vi "Fail interlock.vi"(6 "Select":bool, 7 "Command":T1(ring)=enum."Write task", 8 "error in":errorcluster caption="err out", 9 "Fail Index Out":bool[](array[boolean]), 10 "Inter lock":bool, 11 "Pause":refnum<vi>) -> (0 "error out":errorcluster caption="err out")   [LabVIEW 2016]
uses:
  <vilib>/DAQmx/write.llb/DAQmx Write (Digital Bool 1Line 1Point).vi
  <vilib>/DAQmx/create/channels.llb/DAQmx Create Channel (DO-Digital Output).vi
  <vilib>/DAQmx/miscellaneous.llb/DAQmx Fill In Error Info.vi
panel:
  out "task out":refnum<k21>
  out "Flag":bool=TRUE
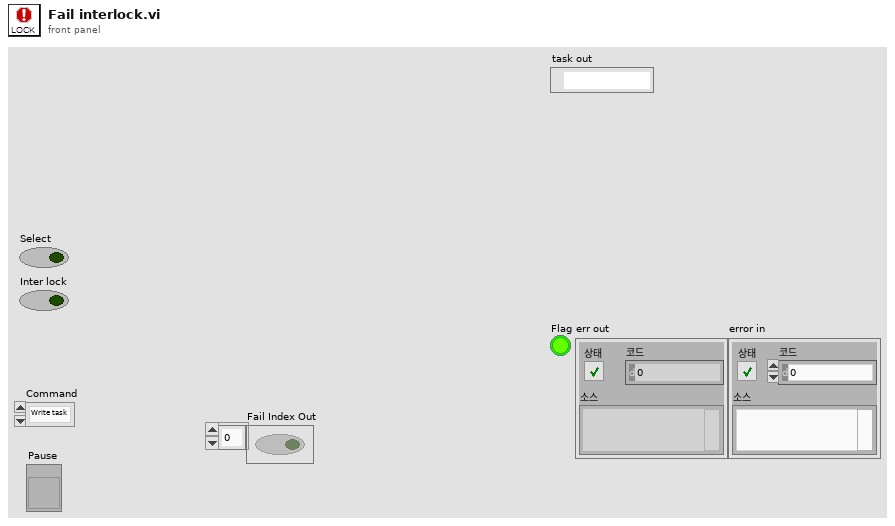
[diagram p1: front panel]
types:
  T1 = enum16{"Flag", "Write task", "Select Data", "Init"}
  T2 = cluster{"Test Information":cluster{"date":string, "custom":string, "oper":string, "package":string, "pkg side":string, "solder":string, "brd side":string, "paste":string, "reflow":string}, "Sensor Set":cluster{"Accelerometer":cluster{"Sensitivity(mV/g)":dbl}, "Strain Guage":cluster{"Ch.":dbl[], "Gage factor":dbl[], "Resistance":dbl[], "Poisson ratio":dbl[]}}, "Resistor Set":cluster{"Criterion Level":dbl, "Res. Set":cluster{"Res. Ch":dbl, "Res. Active":bool, "Res Initial":dbl}[]}, "Test Stop Condition":cluster{"Test cycle":u16, "Fail number in a cycle":u16, "Fail factor":cluster{"Duration":u16, "Fail No.":u16}}, "Acceleration Condition ":cluster{"Shock duration pecent [%]":u16, "Filter cutoff freq":u32}, "Save":cluster{"Save Path":path, "File Name":string}}
  T3 = cluster{"Res. Ch":dbl, "Res. Active":bool, "Res Initial":dbl}[]
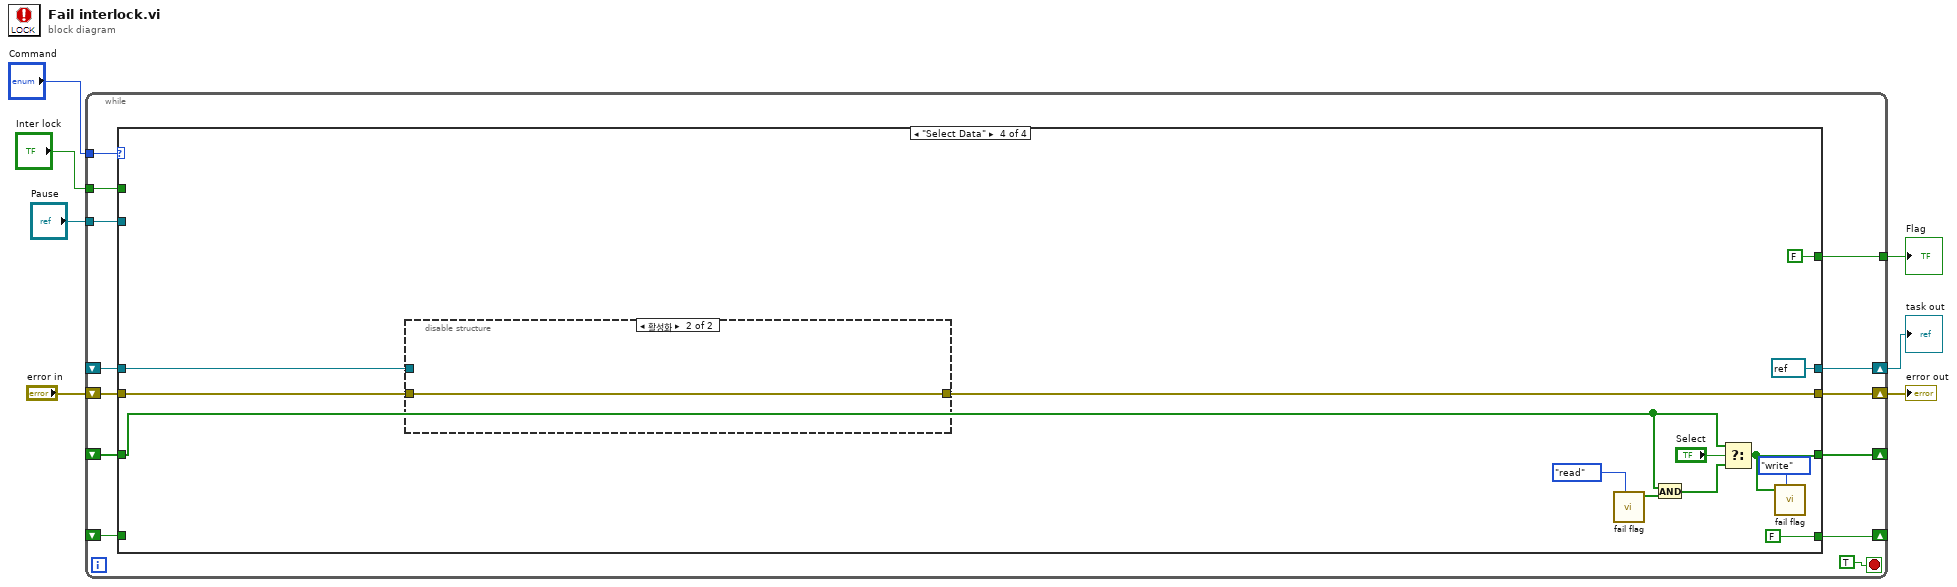
[diagram p0: block diagram]
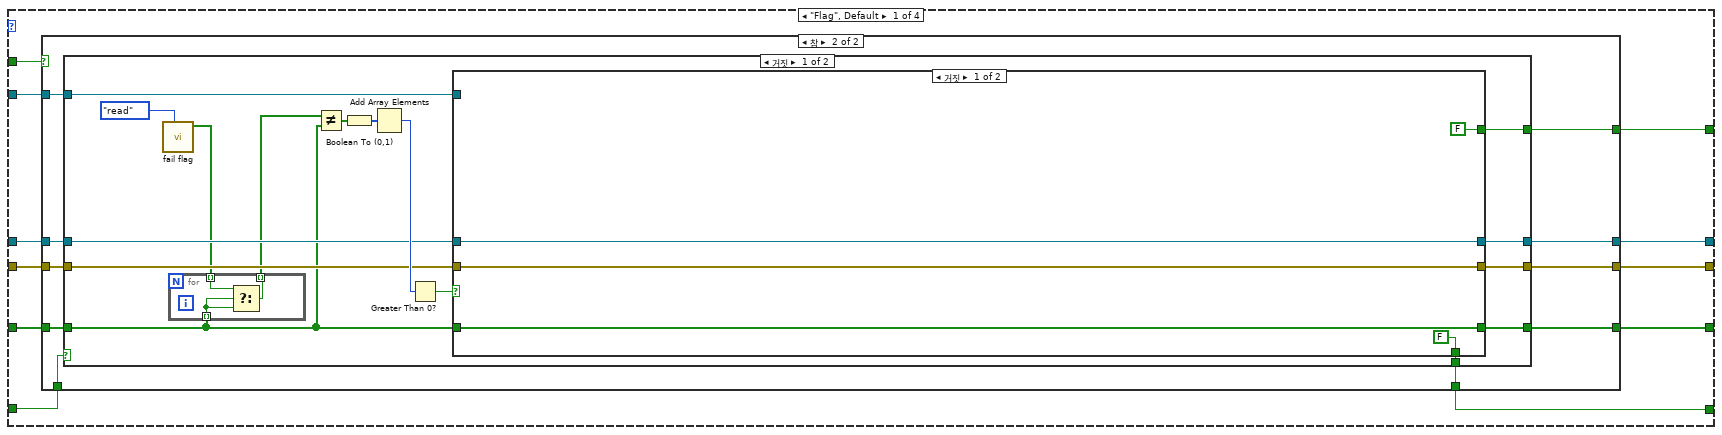
[diagram p2: hidden frame]
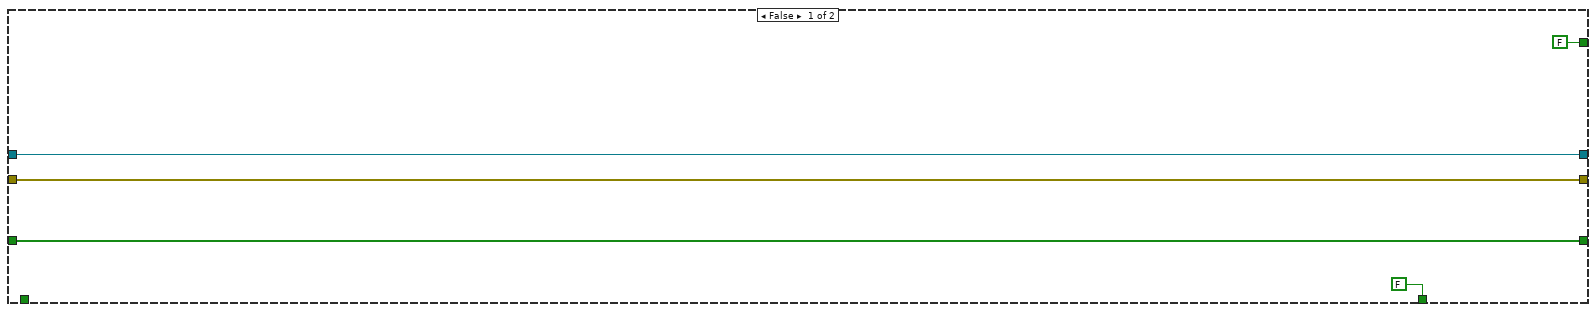
[diagram p3: hidden frame]
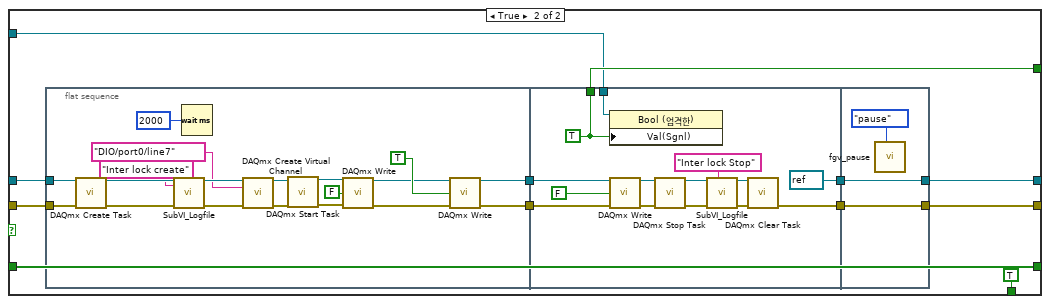
[diagram p4: hidden frame]
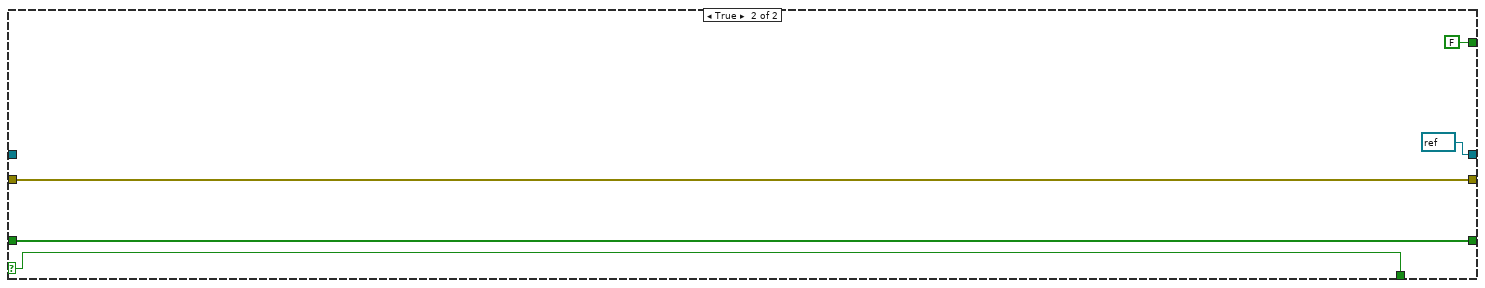
[diagram p5: hidden frame]
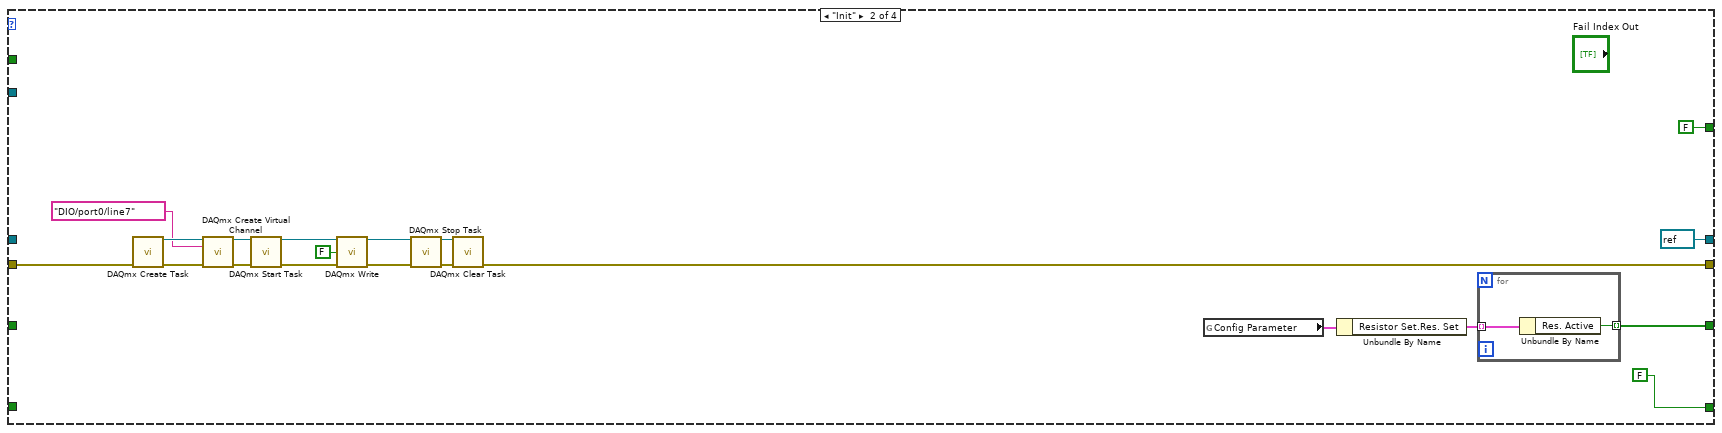
[diagram p6: hidden frame]
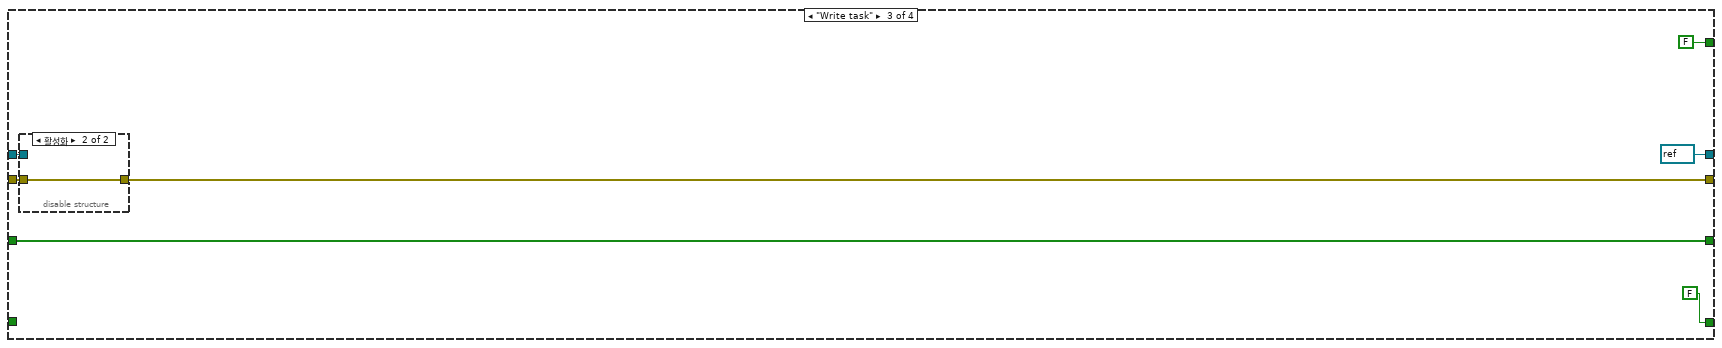
[diagram p7: hidden frame]
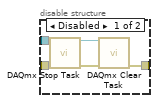
[diagram p8: hidden frame]
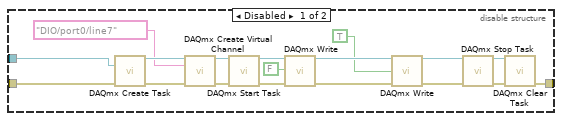
[diagram p9: hidden frame]
diagram:
  n1 = while {
    tunnel: "Command" -> [w19]
    shift-right: [w18] -> _
    shift-left: _ -> [w17]
    tunnel: [w16] -> w6
    tunnel: "Pause" -> [w15]
    shift-right: [w13] -> w1
    shift-left: _ -> [w14]
    shift-right: [w12] -> w4
    shift-left: "error in" -> [w11]
    tunnel: "Inter lock" -> [w10]
    shift-right: [w9] -> _
    shift-left: _ -> [w8]
    stop <- TRUE stop-if-true
    n2 = case shown="\"Select Data\"" w19 {
      tunnel: [w26 w134 w150 w157] -> w18
      tunnel: w17 -> [w27 _ w150 w160]
      tunnel: [w31 FALSE FALSE FALSE] -> w16
      tunnel: w15 -> [w30 _ _ _]
      tunnel: w14 -> [w29 _ w147 w166]
      tunnel: [w28 refnum<k21> refnum ("task out") refnum<k21> refnum ("task out") refnum<k21> refnum ("task out")] -> w13
      tunnel: [w23 w129 w145 w164] -> w12
      tunnel: w11 -> [w24 w137 w146 w165]
      tunnel: w10 -> [w25 _ _ _]
      tunnel: [w22 FALSE FALSE FALSE ("Res. Active")] -> w9
      tunnel: w8 -> [w21 _ _ _]
      frame "Flag", Default {
        n3 = case shown="참" w25 {
          tunnel: [FALSE w46] -> w31
          tunnel: w30 -> [_ w45]
          tunnel: w29 -> [w36 w41]
          tunnel: [w36 w44] -> w28
          tunnel: w27 -> [w35 w43]
          tunnel: [w35 w37] -> w26
          tunnel: w24 -> [w33 w40]
          tunnel: [w33 w42] -> w23
          tunnel: [FALSE w39] -> w22
          tunnel: w21 -> [_ w38]
          frame False {
          }
          frame True {
            n4 = case shown="거짓" w38 {
              selector: w38 -> [_ w118]
              tunnel: [w57 FALSE] -> w46
              tunnel: w45 -> [w56 _]
              tunnel: [w55 refnum<k21> refnum ("task out")] -> w44
              tunnel: w43 -> [w47 w117]
              tunnel: [w54 w119] -> w42
              tunnel: w41 -> [w53 _]
              tunnel: w40 -> [w52 w119]
              tunnel: [w51 w118] -> w39
              tunnel: [w50 w117] -> w37
              frame False {
                n5 = call "fail flag.vi"("Command"=enum16{"init", "read", "write"}."read") -> ("Fail Index Out"=w49:bool[])  [unwired: 10 in]
                n6 = for {
                  tunnel: w47 -> [w63] mode=indexing
                  tunnel: w49 -> [w65] mode=indexing
                  tunnel: [w64] -> w48 mode=indexing
                  n7 = Select(t=w65, s=w63, f=w63) -> (s? t:f=w64:bool)
                }
                n8 = Not Equal?(x=w48, y=w47) -> (x != y?=w61:bool[])
                n9 = Boolean To (0,1)(Boolean=w61) -> (0, 1=w60:i16[])
                n10 = Add Array Elements(numeric array=w60) -> (sum=w59:i16)
                n11 = Greater Than 0?(x=w59) -> (x > 0?=w58:bool)
                n12 = case shown="거짓" w58 {
                  tunnel: [w69 w79] -> w50
                  tunnel: [FALSE w72] -> w57
                  tunnel: w56 -> [_ w71]
                  tunnel: w53 -> [w66 w82]
                  tunnel: [w66 w81] -> w55
                  tunnel: w47 -> [w69 w79]
                  tunnel: w52 -> [w67 w78]
                  tunnel: [w67 w76] -> w54
                  tunnel: [FALSE TRUE] -> w51
                  frame False {
                  }
                  frame True {
                    n13 = flat-sequence {
                      tunnel: w82 -> [w93]
                      tunnel: [w100] -> w80
                      tunnel: w78 -> [w92]
                      tunnel: [w97] -> w77
                      tunnel: w80 -> [w112]
                      tunnel: w77 -> [w109]
                      tunnel: [refnum<k21> refnum ("task out")] -> w74
                      tunnel: [w106] -> w73
                      tunnel: [w105] -> w72
                      tunnel: w71 -> [w104]
                      tunnel: [w115] -> w76
                      tunnel: [w116] -> w81
                      tunnel: w74 -> [w116]
                      tunnel: w73 -> [w115]
                      frame #0 {
                        n14 = call <vilib>:"DAQmx Create Task.vi"("task to copy"=w93, "error in"=w92) -> ("task out"=w96:refnum<k21>, "error out"=w89:errorcluster)  [unwired: 12 in]
                        n15 = call "SubVI_Logfile.vi"("Title"="Inter lock create", "error in"=w89) -> ("error out"=w88:errorcluster)  [unwired: 9 in]
                        n16 = Wait (ms)(milliseconds to wait=u32 2000 ("대기 시간(ms)")) -> ()  [unwired: 1 out]
                        n17 = call-poly <vilib>:"DAQmx Create Virtual Channel.vi"("task in"=w96, "lines"=tag "DIO/port0/line7", "error in"=w88) -> ("task out"=w86:refnum<k21>, "error out"=w84:errorcluster)  [unwired: 11 in]
                        n18 = call <vilib>:"DAQmx Start Task.vi"("task/channels in"=w86, "error in"=w84) -> ("task out"=w85:refnum<k21>, "error out"=w83:errorcluster)  [unwired: 12 in]
                        n19 = call-poly <vilib>:"DAQmx Write.vi"("task/channels in"=w85, "data"=FALSE, "error in"=w83) -> ("task out"=w91:refnum<k21>, "error out"=w90:errorcluster)  [unwired: 10 in, 1 out]
                        n20 = call-poly <vilib>:"DAQmx Write.vi"("task/channels in"=w91, "data"=TRUE, "error in"=w90) -> ("task out"=w100:refnum<k21>, "error out"=w97:errorcluster)  [unwired: 10 in, 1 out]
                      }
                      frame #1 {
                        w105 = TRUE
                        n21 = property class="Bool (엄격한)"(reference=w104, "Val(Sgnl)"=w105) -> ()  [unwired: 1 in, 2 out]
                        n22 = call-poly <vilib>:"DAQmx Write.vi"("task/channels in"=w112, "data"=FALSE, "error in"=w109) -> ("task out"=w111:refnum<k21>, "error out"=w110:errorcluster)  [unwired: 10 in, 1 out]
                        n23 = call <vilib>:"DAQmx Stop Task.vi"("task/channels in"=w111, "error in"=w110) -> ("task out"=w113:refnum<k21>, "error out"=w103:errorcluster)  [unwired: 12 in]
                        n24 = call "SubVI_Logfile.vi"("Title"="Inter lock Stop", "error in"=w103) -> ("error out"=w102:errorcluster)  [unwired: 9 in]
                        n25 = call <vilib>:"DAQmx Clear Task.vi"("task in"=w113, "error in"=w102) -> ("error out"=w106:errorcluster)  [unwired: 13 in]
                      }
                      frame #2 {
                        n26 = call "fgv_pause.vi"("cmd"=enum16{"default", "ini", "pause"}."pause") -> ()  [unwired: 9 in, 2 out]
                      }
                    }
                  }
                }
              }
              frame True {
              }
            }
          }
        }
      }
      frame "Init" {
        n27 = call <vilib>:"DAQmx Create Task.vi"("error in"=w137) -> ("task out"=w140:refnum<k21>, "error out"=w139:errorcluster)  [unwired: 13 in]
        n28 = call-poly <vilib>:"DAQmx Create Virtual Channel.vi"("task in"=w140, "lines"=tag "DIO/port0/line7", "error in"=w139) -> ("task out"=w124:refnum<k21>, "error out"=w123:errorcluster)  [unwired: 11 in]
        n29 = call <vilib>:"DAQmx Start Task.vi"("task/channels in"=w124, "error in"=w123) -> ("task out"=w125:refnum<k21>, "error out"=w122:errorcluster)  [unwired: 12 in]
        n30 = call-poly <vilib>:"DAQmx Write.vi"("task/channels in"=w125, "data"=FALSE, "error in"=w122) -> ("task out"=w128:refnum<k21>, "error out"=w130:errorcluster)  [unwired: 10 in, 1 out]
        n31 = call <vilib>:"DAQmx Stop Task.vi"("task/channels in"=w128, "error in"=w130) -> ("task out"=w132:refnum<k21>, "error out"=w131:errorcluster)  [unwired: 12 in]
        n32 = call <vilib>:"DAQmx Clear Task.vi"("task in"=w132, "error in"=w131) -> ("error out"=w129:errorcluster)  [unwired: 13 in]
        n33 = global read "글로벌_Config Parameter.vi" "Config Parameter"() -> (w136:T2)
        n34 = Unbundle By Name(w136) -> ("Resistor Set.Res. Set"=w135:T3)
        n35 = for {
          tunnel: w135 -> [w143] mode=indexing
          tunnel: [w142] -> w134 mode=indexing
          n36 = Unbundle By Name(w143) -> ("Res. Active"=w142:bool)
        }
      }
      frame "Write task" {
        n37 = disable-structure shown="활성화" {
          disable-tunnel: w147 -> [w153 _]
          disable-tunnel: w146 -> [w152 w156]
          disable-tunnel: [w151 w156] -> w145
          frame Disabled {
            n38 = call <vilib>:"DAQmx Stop Task.vi"("task/channels in"=w153, "error in"=w152) -> ("task out"=w155:refnum<k21>, "error out"=w154:errorcluster)  [unwired: 12 in]
            n39 = call <vilib>:"DAQmx Clear Task.vi"("task in"=w155, "error in"=w154) -> ("error out"=w151:errorcluster)  [unwired: 13 in]
          }
          frame Enabled {
          }
        }
      }
      frame "Select Data" {
        n40 = disable-structure shown="활성화" {
          disable-tunnel: w166 -> [w181 _]
          disable-tunnel: w165 -> [w180 w188]
          disable-tunnel: [w174 w188] -> w164
          frame Disabled {
            n41 = call <vilib>:"DAQmx Create Task.vi"("task to copy"=w181, "error in"=w180) -> ("task out"=w183:refnum<k21>, "error out"=w184:errorcluster)  [unwired: 12 in]
            n42 = call-poly <vilib>:"DAQmx Create Virtual Channel.vi"("task in"=w183, "lines"=tag "DIO/port0/line7", "error in"=w184) -> ("task out"=w172:refnum<k21>, "error out"=w171:errorcluster)  [unwired: 11 in]
            n43 = call <vilib>:"DAQmx Start Task.vi"("task/channels in"=w172, "error in"=w171) -> ("task out"=w173:refnum<k21>, "error out"=w170:errorcluster)  [unwired: 12 in]
            n44 = call-poly <vilib>:"DAQmx Write.vi"("task/channels in"=w173, "data"=FALSE, "error in"=w170) -> ("task out"=w186:refnum<k21>, "error out"=w187:errorcluster)  [unwired: 10 in, 1 out]
            n45 = call-poly <vilib>:"DAQmx Write.vi"("task/channels in"=w186, "data"=TRUE, "error in"=w187) -> ("task out"=w176:refnum<k21>, "error out"=w175:errorcluster)  [unwired: 10 in, 1 out]
            n46 = call <vilib>:"DAQmx Stop Task.vi"("task/channels in"=w176, "error in"=w175) -> ("task out"=w177:refnum<k21>, "error out"=w178:errorcluster)  [unwired: 12 in]
            n47 = call <vilib>:"DAQmx Clear Task.vi"("task in"=w177, "error in"=w178) -> ("error out"=w174:errorcluster)  [unwired: 13 in]
          }
          frame Enabled {
          }
        }
        n48 = call "fail flag.vi"("Command"=enum16{"init", "read", "write"}."read") -> ("Fail Index Out"=w159:bool[])  [unwired: 10 in]
        n49 = And(x=w160, y=w159) -> (x .and. y?=w161:bool[])
        n50 = Select(t=w160, s="Select", f=w161) -> (s? t:f=w157:bool[])
        n51 = call "fail flag.vi"("Command"=enum16{"init", "read", "write"}."write", "Fail Index"=w157) -> ()  [unwired: 9 in, 1 out]
      }
    }
  }
  "Flag" <- w6
  "error out" <- w4
  "task out" <- w1
